vi "E09_FlatSequence.vi"() -> ()   [LabVIEW 2026]
panel:
  out "Boolean 3":bool
  out "Boolean 2":bool
  out "Boolean":bool
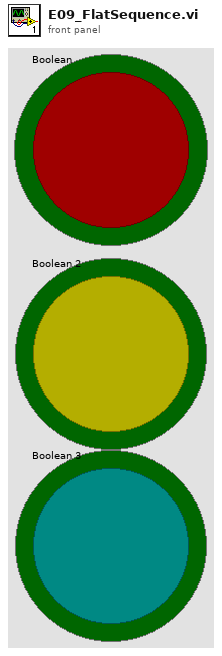
[diagram p1: front panel]
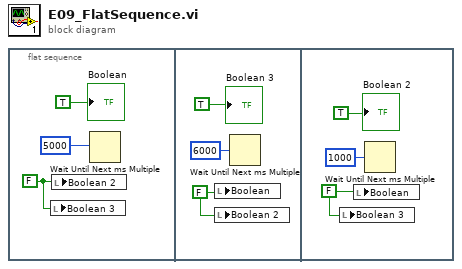
[diagram p0: block diagram]
diagram:
  n1 = flat-sequence {
    frame #0 {
      w1 = FALSE
      n2 = local write "Boolean 3"(w1) -> ()
      n3 = local write "Boolean 2"(w1) -> ()
      n4 = Wait Until Next ms Multiple(millisecond multiple=u32 5000 ("millisecond timer value")) -> ()  [unwired: 1 out]
      "Boolean" <- TRUE
    }
    frame #1 {
      w6 = FALSE
      n5 = local write "Boolean"(w6) -> ()
      n6 = local write "Boolean 2"(w6) -> ()
      n7 = Wait Until Next ms Multiple(millisecond multiple=u32 6000) -> ()  [unwired: 1 out]
      "Boolean 3" <- TRUE
    }
    frame #2 {
      w9 = FALSE
      n8 = local write "Boolean 3"(w9) -> ()
      n9 = local write "Boolean"(w9) -> ()
      n10 = Wait Until Next ms Multiple(millisecond multiple=u32 1000) -> ()  [unwired: 1 out]
      "Boolean 2" <- TRUE
    }
  }
